vi "WLAN - TV - OPPO - RW - UTIL - TestVectors_11B.vi"(0 "TV_IQComposite_11B":T1={"Standard"=0, "DSSS Demod Parameters"={"DSSS Auto Compute Acquisition Length Enabled"=0, "DSSS Equalization Enabled"=0, "DSSS Header Detection Enabled"=0, "DSSS MAC FCS Check Enabled"=0, "DSSS Measurement Start Location"=0, "DSSS Phase Tracking Method"=0, "DSSS Maximum Chips Used"=0, "DSSS Reference Pulse Shaping Filter"=0, "DSSS Reference Pulse Shaping Filter Coefficient"=0.0, "# Avg"=1024, "# Iterations"=1024, "DSSS Power Ramp Enabled"=0}, "Measurement Enabled ? "=FALSE, "Power Level(dBm)"=0.0, "Center Frequency(Hz)"=0.0, "DSSS Generate Parameters"={"DSSS Data Rate (Mbps)"=0, "DSSS Payload Length (bytes)"=1024, "Idle Interval(S)"=0.0}} {"DSSS Generate Parameters"."DSSS Data Rate (Mbps)" items=["1", "2", "5.5 CCK", "5.5 PBCC", "11 CCK", "11 PBCC", "22", "33"]; "Center Frequency(Hz)" format="%#_6p"; "DSSS Demod Parameters"."DSSS Power Ramp Enabled" items=["False", "True"]; "DSSS Demod Parameters"."DSSS Auto Compute Acquisition Length Enabled" items=["False", "True"]; "DSSS Demod Parameters"."DSSS Phase Tracking Method" items=["Standard", "Instantaneous"]; "DSSS Demod Parameters"."DSSS Equalization Enabled" items=["False", "True"]; "DSSS Demod Parameters"."DSSS Reference Pulse Shaping Filter" items=["Rectangular", "Raised Cosine", "Root Raised Cosine", "Gaussian"]; "DSSS Demod Parameters"."DSSS MAC FCS Check Enabled" items=["False", "True"]; "DSSS Demod Parameters"."DSSS Header Detection Enabled" items=["False", "True"]; "Standard" items=["80211A/G/J/P OFDM", "80211B/G DSSS", "80211G DSSSOFDM", "80211N MIMOOFDM", "80211AC MIMOOFDM"]}, 9 "TV Paramaters":T3) -> (6 "TV":string[][](array[string]), 8 "Measure Config":string[][](array[string]))   [LabVIEW 2012]
uses:
  Includes/WLAN - TV - RW - INC - TV_Parameters.ctl
  Includes/WLAN - TV - OPPO - RW - INC - TV_IQComposite_11B.ctl
  Includes/WLAN - TV - RW - INC - TV_DSSS Demod.ctl
  Includes/WLAN - TV - RW - INC - Tx_Meas_Settings_DSSS_String.ctl
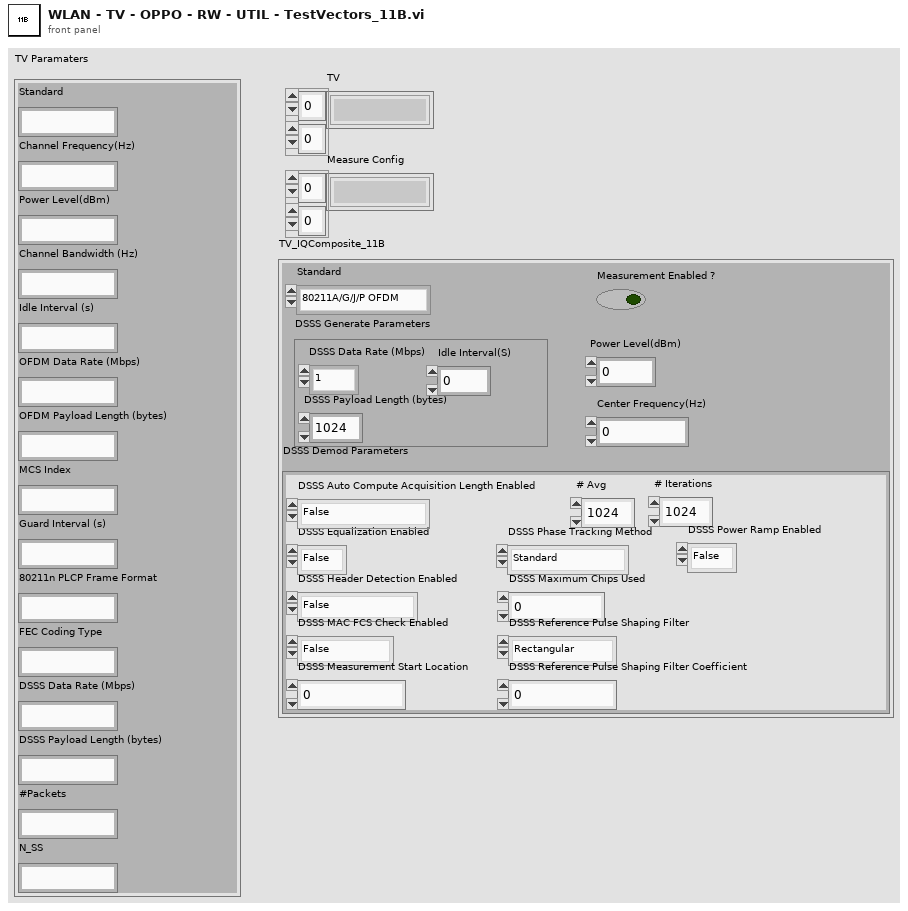
[diagram p1: front panel]
types:
  T1 = typedef "WLAN - TV - OPPO - RW - INC - TV_IQComposite_11B.ctl" = cluster{"Standard":i32, "DSSS Demod Parameters":T2, "Measurement Enabled ? ":bool, "Power Level(dBm)":dbl, "Center Frequency(Hz)":dbl, "DSSS Generate Parameters":cluster{"DSSS Data Rate (Mbps)":i32, "DSSS Payload Length (bytes)":i32, "Idle Interval(S)":dbl}}
  T2 = typedef "WLAN - TV - RW - INC - TV_DSSS Demod.ctl" = cluster{"DSSS Auto Compute Acquisition Length Enabled":i32, "DSSS Equalization Enabled":i32, "DSSS Header Detection Enabled":i32, "DSSS MAC FCS Check Enabled":i32, "DSSS Measurement Start Location":i32, "DSSS Phase Tracking Method":i32, "DSSS Maximum Chips Used":i32, "DSSS Reference Pulse Shaping Filter":i32, "DSSS Reference Pulse Shaping Filter Coefficient":dbl, "# Avg":i32, "# Iterations":i32, "DSSS Power Ramp Enabled":i32}
  T3 = typedef "WLAN - TV - RW - INC - TV_Parameters.ctl" = cluster{"Standard ":string, "Channel Frequency(Hz)":string, "Power Level(dBm)":string, "Channel Bandwidth (Hz)":string, "Idle Interval (s)":string, "OFDM Data Rate (Mbps)":string, "OFDM Payload Length (bytes)":string, "MCS Index":string, "Guard Interval (s)":string, "80211n PLCP Frame Format":string, "FEC Coding Type":string, "DSSS Data Rate (Mbps)":string, "DSSS Payload Length (bytes)":string, "#Packets":string, "N_SS":string}
  T4 = typedef "WLAN - TV - RW - INC - Tx_Meas_Settings_DSSS_String.ctl" = cluster{"DSSS Auto Compute Acquisition Length Enabled":string, "DSSS Equalization Enabled":string, "DSSS Header Detection Enabled":string, "DSSS MAC FCS Check Enabled":string, "DSSS Measurement Start Location":string, "DSSS Phase Tracking Method":string, "DSSS Maximum Chips Used":string, "DSSS Reference Pulse Shaping Filter":string, "DSSS Reference Pulse Shaping Filter Coefficient":string, "#Avg":string, "#Iterations":string, "DSSS Ramp Enabled ":string}
  T5 = cluster{"DSSS Data Rate (Mbps)":i32, "DSSS Payload Length (bytes)":i32, "Idle Interval(S)":dbl}
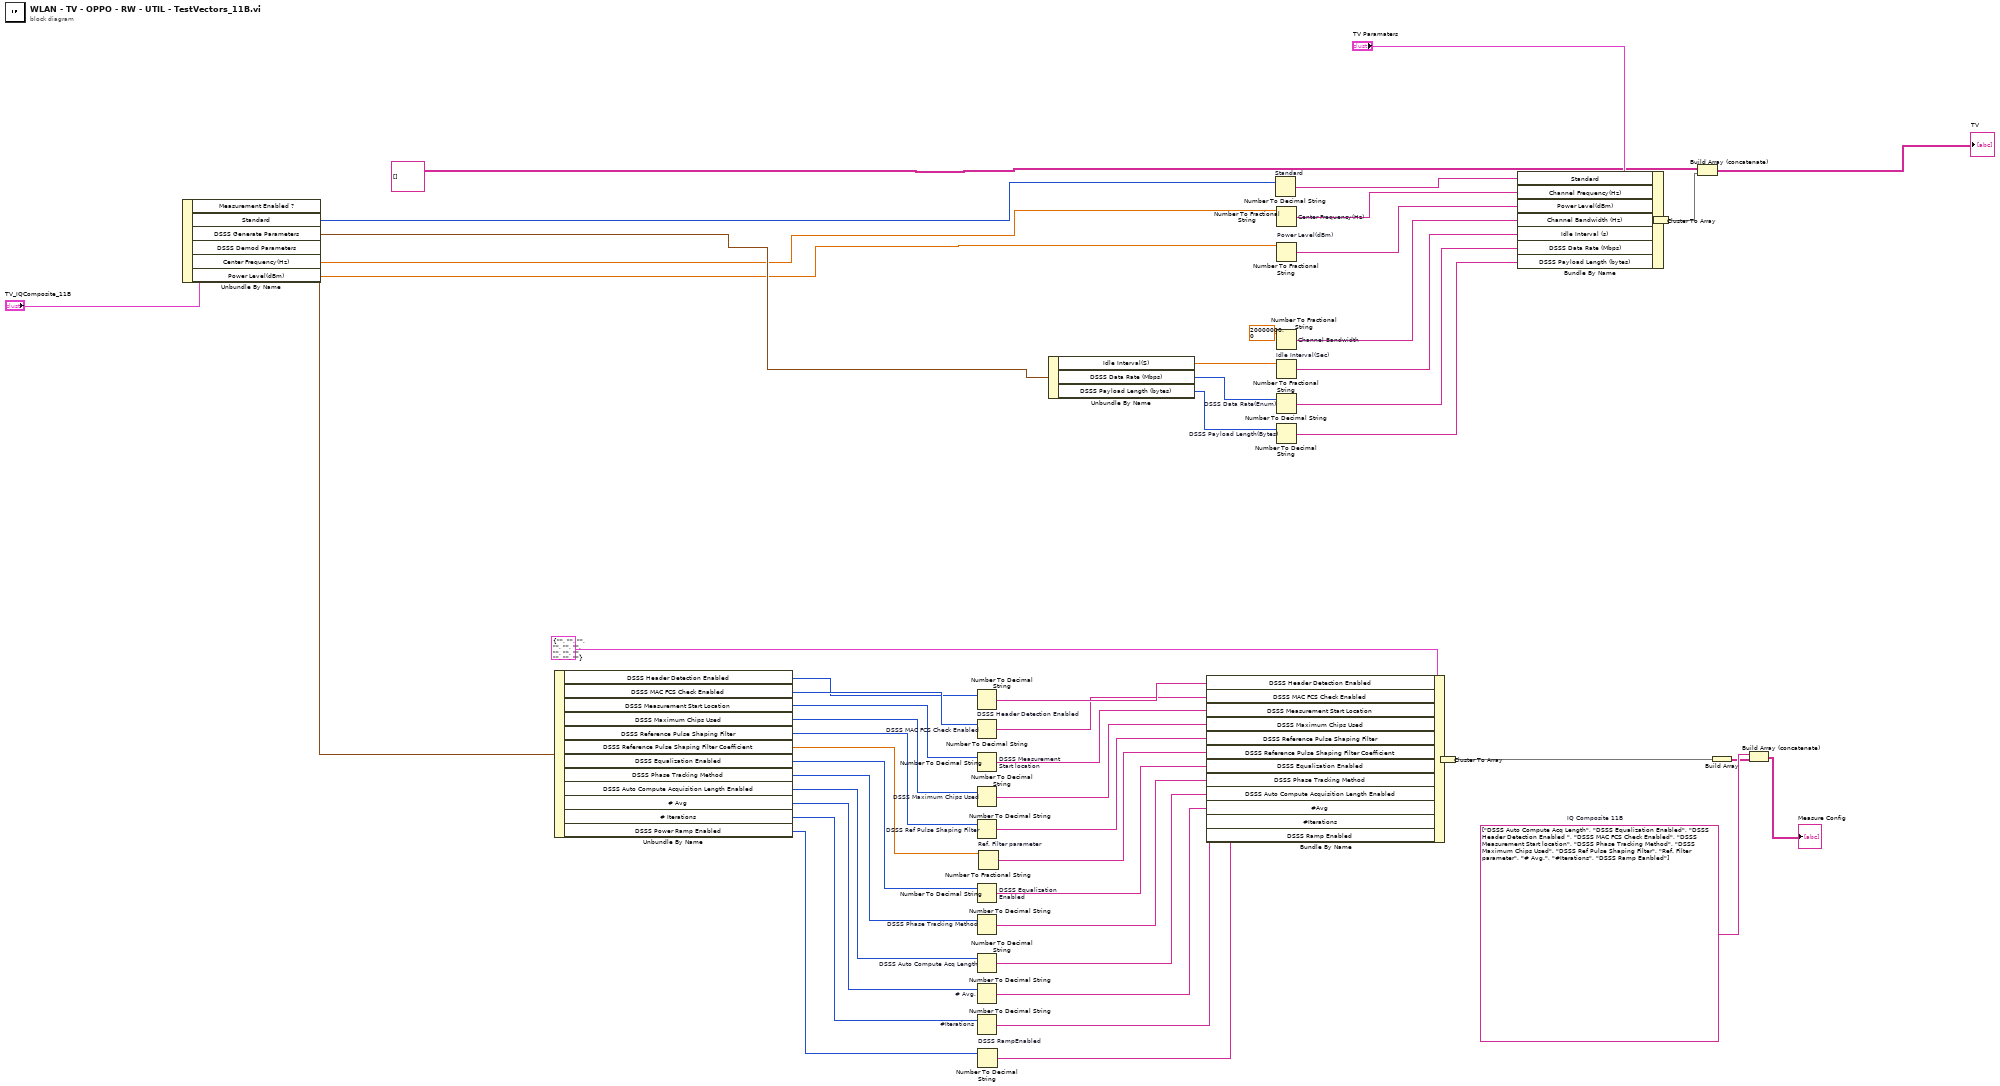
[diagram p0: block diagram]
diagram:
  w28 = string[] ["DSSS Auto Compute Acq Length", "DSSS Equalization Enabled", "DSSS Header Detection Enabled ", "DSSS MAC FCS Check Enabled", "DSSS Measurement Start location", "DSSS Phase Tracking Method", "DSSS Maximum Chips Used", "DSSS Ref Pulse Shaping Filter", "Ref. Filter parameter", "# Avg.", "#Iterations", "DSSS Ramp Eanbled"]  # IQ Composite 11B
  n1 = Unbundle By Name("TV_IQComposite_11B") -> ("Standard"=w51:i32, "DSSS Generate Parameters"=w52:T5, "DSSS Demod Parameters"=w26:T2, "Center Frequency(Hz)"=w15:dbl, "Power Level(dBm)"=w14:dbl)  [unwired: 1 out]
  n2 = Unbundle By Name(w26) -> ("DSSS Header Detection Enabled"=w39:i32, "DSSS MAC FCS Check Enabled"=w40:i32, "DSSS Measurement Start Location"=w41:i32, "DSSS Maximum Chips Used"=w42:i32, "DSSS Reference Pulse Shaping Filter"=w43:i32, "DSSS Reference Pulse Shaping Filter Coefficient"=w24:dbl, "DSSS Equalization Enabled"=w44:i32, "DSSS Phase Tracking Method"=w45:i32, "DSSS Auto Compute Acquisition Length Enabled"=w46:i32, "# Avg"=w47:i32, "# Iterations"=w48:i32, "DSSS Power Ramp Enabled"=w23:i32)
  n3 = Number To Decimal String "DSSS Header Detection Enabled"(number=w39) -> (decimal integer string=w38:string)  [unwired: 1 in]
  n4 = Number To Decimal String "DSSS MAC FCS Check Enabled"(number=w40) -> (decimal integer string=w37:string)  [unwired: 1 in]
  n5 = Number To Decimal String "DSSS Measurement Start location"(number=w41) -> (decimal integer string=w36:string)  [unwired: 1 in]
  n6 = Number To Decimal String "DSSS Maximum Chips Used"(number=w42) -> (decimal integer string=w35:string)  [unwired: 1 in]
  n7 = Number To Decimal String "DSSS Ref Pulse Shaping Filter"(number=w43) -> (decimal integer string=w34:string)  [unwired: 1 in]
  n8 = Number To Decimal String "DSSS Equalization Enabled"(number=w44) -> (decimal integer string=w29:string)  [unwired: 1 in]
  n9 = Number To Decimal String "DSSS Phase Tracking Method"(number=w45) -> (decimal integer string=w30:string)  [unwired: 1 in]
  n10 = Number To Decimal String "DSSS Auto Compute Acq Length"(number=w46) -> (decimal integer string=w31:string)  [unwired: 1 in]
  n11 = Number To Decimal String "# Avg."(number=w47) -> (decimal integer string=w32:string)  [unwired: 1 in]
  n12 = Number To Decimal String "#Iterations"(number=w48) -> (decimal integer string=w33:string)  [unwired: 1 in]
  n13 = Number To Decimal String "DSSS RampEnabled"(number=w23) -> (decimal integer string=w22:string)  [unwired: 1 in]
  n14 = Number To Fractional String "Ref. Filter parameter"(number=w24) -> (F-format string=w25:string)  [unwired: 3 in]
  n15 = Unbundle By Name(w52) -> ("Idle Interval(S)"=w3:dbl, "DSSS Data Rate (Mbps)"=w5:i32, "DSSS Payload Length (bytes)"=w4:i32)
  n16 = Bundle By Name(cluster=T4 {"DSSS Auto Compute Acquisition Length Enabled"="", "DSSS Equalization Enabled"="", "DSSS Header Detection Enabled"="", "DSSS MAC FCS Check Enabled"="", "DSSS Measurement Start Location"="", "DSSS Phase Tracking Method"="", "DSSS Maximum Chips Used"="", "DSSS Reference Pulse Shaping Filter"="", "DSSS Reference Pulse Shaping Filter Coefficient"="", "#Avg"="", "#Iterations"="", "DSSS Ramp Enabled "=""} ("OFDM Measurement Settings"), "DSSS Header Detection Enabled"=w38, "DSSS MAC FCS Check Enabled"=w37, "DSSS Measurement Start Location"=w36, "DSSS Maximum Chips Used"=w35, "DSSS Reference Pulse Shaping Filter"=w34, "DSSS Reference Pulse Shaping Filter Coefficient"=w25, "DSSS Equalization Enabled"=w29, "DSSS Phase Tracking Method"=w30, "DSSS Auto Compute Acquisition Length Enabled"=w31, "#Avg"=w32, "#Iterations"=w33, "DSSS Ramp Enabled"=w22) -> (w21:T4)
  n17 = Number To Decimal String "Standard"(number=w51) -> (decimal integer string=w6:string)  [unwired: 1 in]
  n18 = Number To Fractional String "Center Frequency(Hz)"(number=w15) -> (F-format string=w7:string)  [unwired: 3 in]
  n19 = Number To Fractional String "Power Level(dBm)"(number=w14) -> (F-format string=w8:string)  [unwired: 3 in]
  n20 = Number To Fractional String "Channel Bandwidth"(number=20000000.0) -> (F-format string=w9:string)  [unwired: 3 in]
  n21 = Number To Fractional String "Idle Interval(Sec)"(number=w3) -> (F-format string=w10:string)  [unwired: 3 in]
  n22 = Number To Decimal String "DSSS Data Rate(Enum)"(number=w5) -> (decimal integer string=w11:string)  [unwired: 1 in]
  n23 = Number To Decimal String "DSSS Payload Length(Bytes)"(number=w4) -> (decimal integer string=w12:string)  [unwired: 1 in]
  n24 = Cluster To Array(cluster=w21) -> (array=w20:string[])
  n25 = Bundle By Name(cluster="TV Paramaters", "Standard"=w6, "Channel Frequency(Hz)"=w7, "Power Level(dBm)"=w8, "Channel Bandwidth (Hz)"=w9, "Idle Interval (s)"=w10, "DSSS Data Rate (Mbps)"=w11, "DSSS Payload Length (bytes)"=w12) -> (w2:T3)
  n26 = Cluster To Array(cluster=w2) -> (array=w1:string[])
  n27 = Build Array (concatenate)(string[][] [] ("appended array"), w1) -> (→"TV":string[][])
  n28 = Build Array(w20) -> (w27:string[][])
  n29 = Build Array (concatenate)(w28, w27) -> (→"Measure Config":string[][])
